vi "authorize calculate action.vi"(2 "Content (\"\")":string, 3 "Query Params":T1) -> (0 "Action":string, 1 "Query Params":T1)   [LabVIEW 2011]
uses:
  ITK EXT/utils/keyedarr.llb/Keyed Array.ctl
  ITK EXT/utils/strutil.llb/Case Matching.ctl
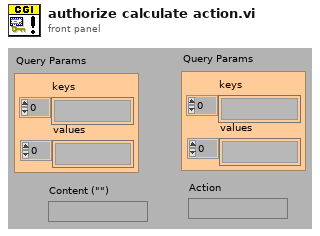
[diagram p1: front panel]
types:
  T1 = typedef "Keyed Array.ctl" = cluster{"keys":string[], "values":string[]}
  T2 = typedef "Case Matching.ctl" = enum16{"a != A", "a == A", "system"}
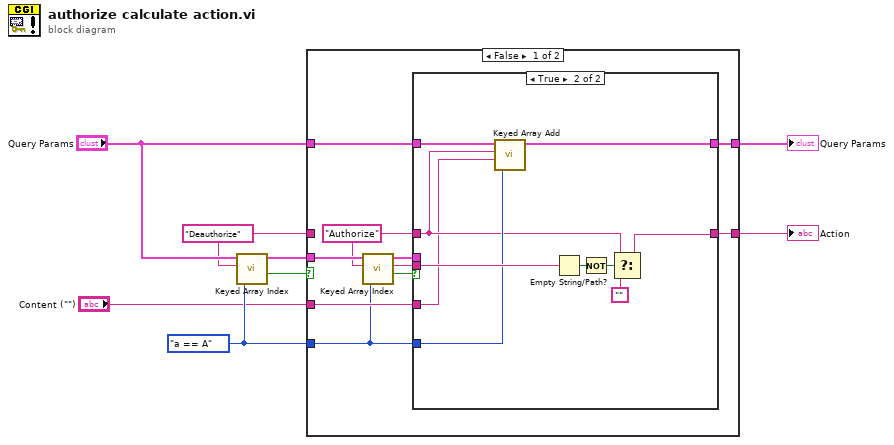
[diagram p0: block diagram]
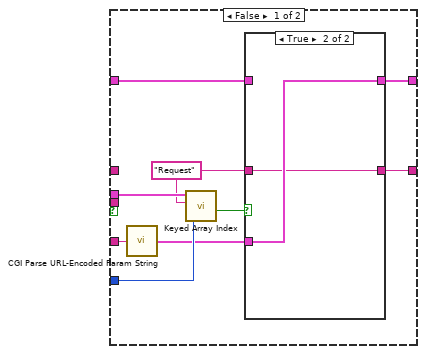
[diagram p2: hidden frame]
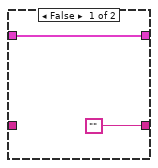
[diagram p3: hidden frame]
diagram:
  w1 = "Deauthorize"
  w3 = Case_Matching."a == A" ("case matching (sensitive)")
  n1 = call "Keyed Array Index.vi"("case matching (sensitive)"=w3, "key"=w1, "array in"="Query Params") -> ("valid key"=w6:bool, "duplicate array"=w7:T1)  [unwired: 1 in, 2 out]
  n2 = case shown="False" w6 {
    tunnel: w1 -> [_ w43]
    tunnel: [w13 w43] -> w8
    tunnel: w7 -> [w18 _]
    tunnel: w3 -> [w11 _]
    tunnel: "Query Params" -> [w15 w42]
    tunnel: [w14 w42] -> w4
    tunnel: "Content (\"\")" -> [w12 _]
    frame False {
      w9 = "Authorize"
      n3 = call "Keyed Array Index.vi"("case matching (sensitive)"=w11, "key"=w9, "array in"=w18) -> ("valid key"=w17:bool, "value"=w16:string, "duplicate array"=w10:T1)  [unwired: 1 in, 1 out]
      n4 = case shown="True" w17 {
        tunnel: w16 -> [_ w41]
        tunnel: w9 -> [_ w33]
        tunnel: w15 -> [w25 w36]
        tunnel: [w24 w35] -> w14
        tunnel: [w23 w39] -> w13
        tunnel: w12 -> [w27 w32]
        tunnel: w11 -> [w26 w34]
        tunnel: w10 -> [w21 _]
        frame False {
          w19 = "Request"
          n5 = call "CGI Parse URL-Encoded Param String.vi"("url-encoded param string"=w27) -> ("params"=w20:T1)
          n6 = call "Keyed Array Index.vi"("case matching (sensitive)"=w26, "key"=w19, "array in"=w21) -> ("valid key"=w22:bool)  [unwired: 1 in, 3 out]
          n7 = case shown="True" w22 {
            tunnel: w25 -> [w29 _]
            tunnel: [w29 w31] -> w24
            tunnel: ["" w30] -> w23
            tunnel: w20 -> [_ w31]
            tunnel: w19 -> [_ w30]
            frame False {
            }
            frame True {
            }
          }
        }
        frame True {
          n8 = call "Keyed Array Add.vi"("case matching (sensitive)"=w34, "value"=w32, "key"=w33, "array in"=w36) -> ("array out"=w35:T1)  [unwired: 3 out]
          n9 = Empty String/Path?(string/path=w41) -> (empty?=w40:bool)
          n10 = Not(x=w40) -> (.not. x?=w38:bool)
          n11 = Select(t=w33, s=w38, f="") -> (s? t:f=w39:string)
        }
      }
    }
    frame True {
    }
  }
  "Action" <- w8
  "Query Params" <- w4
